vi "init_pass_buoys.vi"(10 "Buoy Pass 2":cluster{"X":dbl, "Y":dbl}, 11 "Buoy Pass 1":cluster{"X":dbl, "Y":dbl}) -> (2 "Mission.lvclass":refnum<class "Mission.lvclass">)   [LabVIEW 2011, in "Mission.lvclass"]
uses:
  Mission.lvclass
panel:
  in  "Mission out":refnum<class "Mission.lvclass">
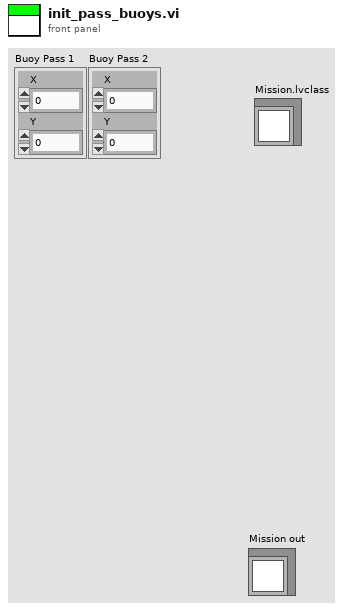
[diagram p1: front panel]
types:
  T1 = enum16{"Round Buoy", "Pass Buoys", "Station Keeping"}
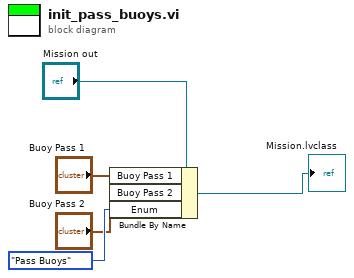
[diagram p0: block diagram]
diagram:
  n1 = Bundle By Name(cluster="Mission out", "Buoy Pass 1"="Buoy Pass 1", "Buoy Pass 2"="Buoy Pass 2", "Enum"=T1."Pass Buoys") -> (→"Mission.lvclass":refnum<class "Mission.lvclass">)
